vi "onProcessKilled.vi"(11 "SMO in":refnum<class "SMO.lvclass">) -> ()   [LabVIEW 2021, in "smo.lvlib" / "SMO.lvclass"]
uses:
  SMO.lvclass
  SMO.lvclass/SMO.ctl
panel:
  # "This method is called if the call chain of the SMO\nis leaving memory while the process is running.\nAssume all references created in caller's thread to\nbe invalid."
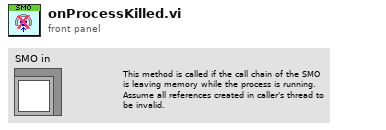
[diagram p1: front panel]
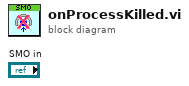
[diagram p0: block diagram]
diagram:
